vi "Map Table.vi"(8 "error in":errorcluster, 9 "Inital Index":i32=1, 11 "picture":refnum<vi>) -> (0 "error out":errorcluster, 5 "picture":picture)   [LabVIEW 2013]
uses:
  Baxter Examples/Arm Globals.vi
  ROS/Code/SubVIs/BaxterSide.ctl
  Prim/Fwd Kenimatics - array.vi
  <vilib>/Analysis/Matrix/NI_Matrix.lvlib
  <vilib>/Analysis/Matrix/Numeric/Multiply/Multiply - RM,RM.vi
  <vilib>/Analysis/Matrix/Datatypes/RealMatrix.ctl
  <vilib>/Analysis/NI_AALBase.lvlib
  <vilib>/Analysis/baseanly.llb/Mean (DBL).vi
  Move Relative XYZRPY.vi
panel:
  # "0:Far Left\n1:Far Right\n2:Near Left\n3:Near Right"
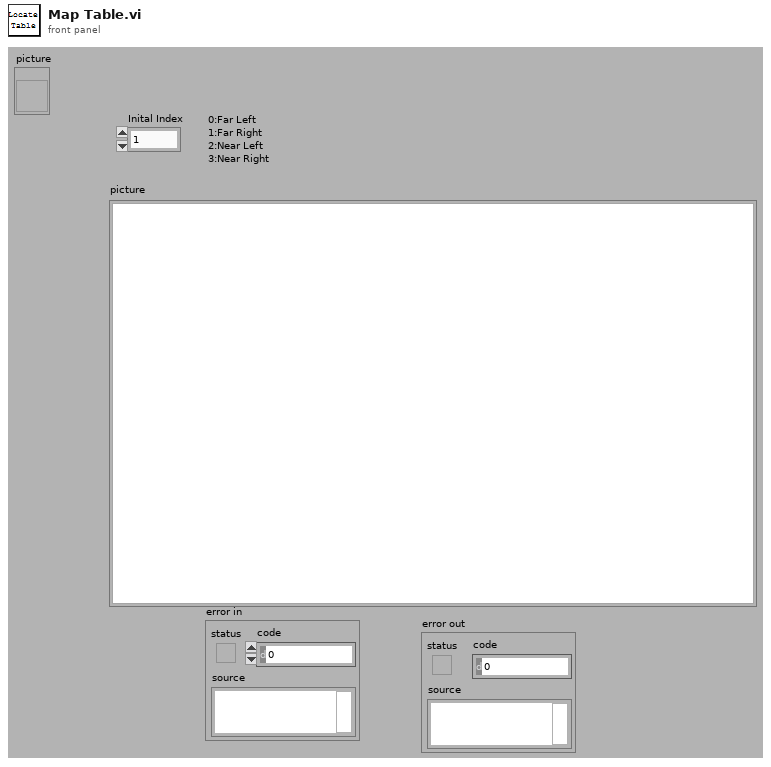
[diagram p1: front panel]
types:
  T1 = typedef "NI_Matrix.lvlib/RealMatrix.ctl" = dbl[][]
  T2 = cluster{"Label":string, "Joints":dbl[], "T":T1}[]
  T3 = typedef "BaxterSide.ctl" = enum16{"left", "right"}
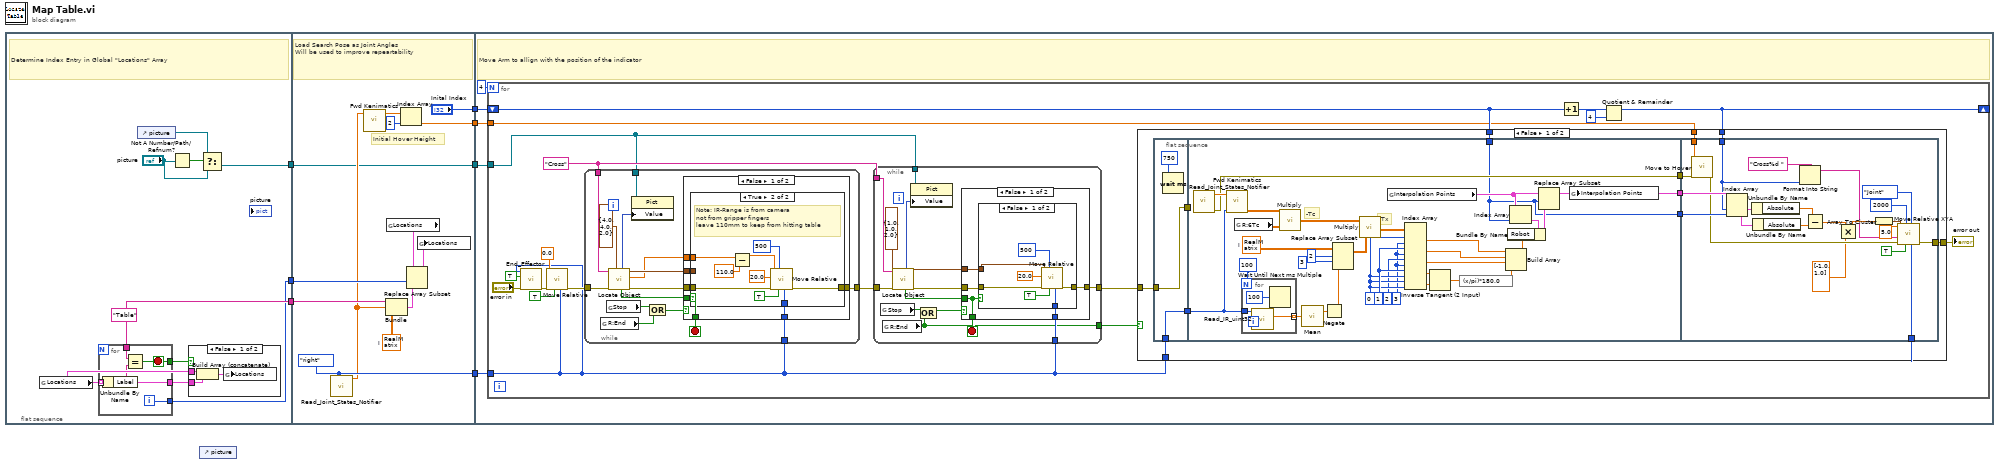
[diagram p0: block diagram]
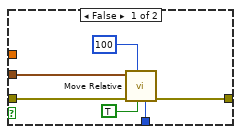
[diagram p6: hidden frame]
diagram:
  n1 = flat-sequence {
    tunnel: [w14] -> w6
    tunnel: [w16] -> w5
    tunnel: [w8] -> w1
    tunnel: [w37] -> w7
    tunnel: w6 -> [w28]
    tunnel: w5 -> [w27]
    tunnel: ["Inital Index"] -> w4
    tunnel: [w33] -> w3
    tunnel: [w25] -> w2
    tunnel: w1 -> [w25]
    tunnel: w7 -> [w42]
    tunnel: w4 -> [w40]
    tunnel: w3 -> [w39]
    tunnel: w2 -> [w38]
    frame #0 {
      w16 = "Table"
      # "Determine Index Entry in Global \"Locations\" Array"
      n2 = global read "Arm Globals.vi" "Locations"() -> (w12:T2)
      n3 = for {
        tunnel: w12 -> [w20] mode=indexing
        tunnel: w16 -> [w23]
        tunnel: [w22] -> w14
        tunnel: [w21] -> w15
        tunnel: [w20] -> w13
        i -> [w22]
        stop <- w21 stop-if-true
        n4 = Unbundle By Name(w20) -> ("Label"=w24:string)
        n5 = Equal?(x=w23, y=w24) -> (x = y?=w21:bool)
      }
      n6 = control-ref of="picture"() -> (w9:refnum<vi>)
      n7 = Not A Number/Path/Refnum?(number/path/refnum="picture") -> (NaN/Path/Refnum?=w11:bool)
      n8 = case shown="False" w15 {
        tunnel: w13 -> [w18 _]
        tunnel: w12 -> [w17 _]
        frame False {
          n9 = Build Array (concatenate)(w17, w18) -> (w19:T2)
          n10 = global write "Arm Globals.vi" "Locations"(w19) -> ()
        }
        frame True {
        }
      }
      n11 = Select(t=w9, s=w11, f="picture") -> (s? t:f=w8:refnum<vi>)
    }
    frame #1 {
      w31 = T1 [[1.0, 0.0, 0.0, 0.0], [0.0, 1.0, 0.0, 0.0], [0.0, 0.0, 1.0, 0.0], [0.0, 0.0, 0.0, 1.0]]  # I
      w37 = BaxterSide."right" ("Side")
      # "Initial Hover Height"
      # "Load Search Pose as Joint Angles\nWill be used to improve repeartability"
      n12 = call "Read_Joint_States_Notifier.vi"("Side"=w37) -> ("Positions"=w26:dbl[])  [unwired: 6 in, 1 out]
      n13 = call-poly "Fwd Kenimatics.vi"("Joints"=w26) -> ("Position"=w35:dbl[])  [unwired: 9 in, 1 out]
      n14 = Bundle(w27, "Positions"=w26, "I"=w31) -> (w32:cluster{string, "Positions":dbl[], "I":T1})  [unwired: 1 in]
      n15 = global read "Arm Globals.vi" "Locations"() -> (w30:T2)
      n16 = Index Array(array=w35, index=2) -> (element=w33:dbl)
      n17 = Replace Array Subset(array=w30, new element=w32, index=w28) -> (w29:T2)
      n18 = global write "Arm Globals.vi" "Locations"(w29) -> ()
    }
    frame #2 {
      # "Move Arm to allign with the position of the indicator"
      n19 = for {
        N: 4 -> [_]
        tunnel: w42 -> [w46]
        shift-right: [w47] -> _
        shift-left: w40 -> [w49]
        tunnel: w39 -> [w48]
        tunnel: w38 -> [w44]
        w55 = "Cross"
        n20 = call "End_Effector.vi"("error in"="error in", "Open"=TRUE, "Side"=w46) -> ("error out"=w58:errorcluster)  [unwired: 5 in]
        n21 = call-poly "Move Relative.vi"("Side"=w46, "Make Vertical"=TRUE, "error in"=w58, "Label"=0.0 ("Z")) -> ("error out"=w57:errorcluster)  [unwired: 7 in]
        n22 = while {
          tunnel: w57 -> [w176]
          tunnel: [w174] -> w60
          tunnel: w55 -> [w171]
          tunnel: w46 -> [w170]
          tunnel: w44 -> [w165]
          stop <- w168 stop-if-true
          n23 = global read "Arm Globals.vi" "R:End"() -> (w166:bool)
          n24 = global read "Arm Globals.vi" "Stop"() -> (w172:bool)
          n25 = call "Locate Object.vi"("Tolerance"=cluster{"x":dbl, "y":dbl, "a":dbl} {"x"=4.0, "y"=4.0, "a"=2.0}, "error in"=w176, "Object"=w171) -> ("error out"=w175:errorcluster, "Range"=w162:dbl, "result"=w173:cluster{"x":dbl, "y":dbl, "a":dbl}, "Close"=w167:bool, "picture"=w163:picture)  [unwired: 3 in, 1 out]
          n26 = property class="Pict"(reference=w165, "Value"=w163) -> ()  [unwired: 1 in, 2 out]
          n27 = Compound Arithmetic op=OR(w172, w166) -> (w169:bool)
          n28 = case shown="False" w169 {
            selector: w169 -> [_ w198]
            tunnel: w175 -> [w182 w199]
            tunnel: [w181 w199] -> w174
            tunnel: w173 -> [w180 _]
            tunnel: w170 -> [w179 _]
            tunnel: [w178 w198] -> w168
            tunnel: w167 -> [w178 _]
            tunnel: w162 -> [w177 _]
            frame False {
              n29 = case shown="True" w178 {
                tunnel: w182 -> [w188 w196]
                tunnel: [w187 w195] -> w181
                tunnel: w180 -> [w184 _]
                tunnel: w179 -> [w186 w194]
                tunnel: w177 -> [_ w190]
                frame False {
                  n30 = call-poly "Move Relative.vi"("Side"=w186, "Make Vertical"=TRUE, "wait time"=100, "error in"=w188, "Goal"=w184) -> ("error out"=w187:errorcluster)  [unwired: 6 in]
                }
                frame True {
                  # "Note: IR-Range is from camera \nnot from gripper fingers\nleave 110mm to keep from hitting table"
                  n31 = Subtract(x=w190, y=110.0) -> (x-y=w189:dbl)
                  n32 = call-poly "Move Relative.vi"("Side"=w194, "Make Vertical"=TRUE, "wait time"=500, "error in"=w196, "Label"=20.0 ("Speed"), "XYZOAT"=w189) -> ("error out"=w195:errorcluster)  [unwired: 5 in]
                }
              }
            }
            frame True {
            }
          }
        }
        n33 = while {
          tunnel: w60 -> [w146]
          tunnel: [w144] -> w52
          tunnel: w55 -> [w141]
          tunnel: w46 -> [w140]
          tunnel: w44 -> [w136]
          tunnel: [w133] -> w43
          stop <- w137 stop-if-true
          n34 = global read "Arm Globals.vi" "Stop"() -> (w142:bool)
          n35 = global read "Arm Globals.vi" "R:End"() -> (w133:bool)
          n36 = call "Locate Object.vi"("Tolerance"=cluster{"x":dbl, "y":dbl, "a":dbl} {"x"=1.0, "y"=1.0, "a"=2.0}, "error in"=w146, "Object"=w141) -> ("error out"=w145:errorcluster, "result"=w143:cluster{"x":dbl, "y":dbl, "a":dbl}, "Close"=w138:bool, "picture"=w134:picture)  [unwired: 3 in, 2 out]
          n37 = property class="Pict"(reference=w136, "Value"=w134) -> ()  [unwired: 1 in, 2 out]
          n38 = Compound Arithmetic op=OR(w142, w133) -> (w139:bool)
          n39 = case shown="False" w139 {
            selector: w139 -> [_ w160]
            tunnel: w138 -> [w147 _]
            tunnel: w145 -> [w151 w161]
            tunnel: [w150 w161] -> w144
            tunnel: w143 -> [w149 _]
            tunnel: w140 -> [w148 _]
            tunnel: [w147 w160] -> w137
            frame False {
              n40 = case shown="False" w147 {
                tunnel: w151 -> [w158 w159]
                tunnel: [w157 w159] -> w150
                tunnel: w149 -> [w154 _]
                tunnel: w148 -> [w156 _]
                frame False {
                  n41 = call-poly "Move Relative.vi"("Side"=w156, "Make Vertical"=TRUE, "wait time"=500, "error in"=w158, "Label"=20.0 ("Speed"), "XYZOAT"=w154) -> ("error out"=w157:errorcluster)  [unwired: 5 in]
                }
                frame True {
                }
              }
            }
            frame True {
            }
          }
        }
        n42 = Increment(x=w49) -> (x+1=w51:i32)
        n43 = Quotient & Remainder(x=w51, y=4) -> (x-y*floor(x/y)=w47:i32)  [unwired: 1 out]
        n44 = case shown="False" w43 {
          tunnel: w52 -> [w66 w132]
          tunnel: w49 -> [w65 _]
          tunnel: w48 -> [w64 _]
          tunnel: w47 -> [w63 _]
          tunnel: w46 -> [w62 _]
          tunnel: [w61 w132] -> w45
          frame False {
            n45 = flat-sequence {
              tunnel: w66 -> [w74]
              tunnel: w62 -> [w73]
              tunnel: [w74] -> w71
              tunnel: [w73] -> w70
              tunnel: w71 -> [_]
              tunnel: w70 -> [w78]
              tunnel: w65 -> [w75]
              tunnel: [w77] -> w69
              tunnel: [w76] -> w68
              tunnel: [w75] -> w67
              tunnel: w64 -> [w131]
              tunnel: w69 -> [w130]
              tunnel: w68 -> [w128]
              tunnel: w63 -> [w118]
              tunnel: w67 -> [w127]
              tunnel: w62 -> [w122]
              tunnel: [w119] -> w61
              frame #0 {
                n46 = Wait (ms)(milliseconds to wait=u32 750) -> ()  [unwired: 1 out]
              }
              frame #1 {
                w97 = 1 ("index (row)")
                w92 = 3 ("index (col)")
                w96 = 0 ("index (row)")
                w86 = T1 [[1.0, 0.0, 0.0, 0.0], [0.0, 1.0, 0.0, 0.0], [0.0, 0.0, 1.0, 0.0], [0.0, 0.0, 0.0, 1.0]]  # I
                # "-Tx"
                # "-Tc"
                n47 = call "Read_Joint_States_Notifier.vi"() -> ("error out"=w77:errorcluster, "Positions"=w79:dbl[])  [unwired: 7 in]
                n48 = call-poly "Fwd Kenimatics.vi"("Side"=w78, "Joints"=w79) -> ("Matrix"=w82:T1)  [unwired: 8 in, 1 out]
                n49 = global read "Arm Globals.vi" "R:6Tc"() -> (w81:T1)
                n50 = for {
                  N: 100 -> [_]
                  tunnel: w78 -> [w109]
                  tunnel: [w108] -> w84 mode=indexing
                  n51 = call "Read_IR_uint32.vi"("Side"=w109) -> ("Distance"=w108:dbl)  [unwired: 4 in, 3 out]
                  n52 = Wait Until Next ms Multiple(millisecond multiple=u32 100) -> ()  [unwired: 1 out]
                }
                n53 = call-poly <vilib>:"Multiply.vi"("Real Matrix B"=w81, "Real Matrix A"=w82) -> ("A * B"=w89:T1)
                n54 = call-poly <vilib>:"Mean.vi"("X"=w84) -> ("mean"=w83:dbl)  [unwired: 1 out]
                n55 = Negate(x=w83) -> (-x=w88:dbl)
                n56 = Replace Array Subset(array=w86, new element=w88, index (row)=2 ("disabled index (row)"), index (col)=3 ("disabled index (col)")) -> (w90:T1)
                n57 = call-poly <vilib>:"Multiply.vi"("Real Matrix B"=w90, "Real Matrix A"=w89) -> ("A * B"=w91:T1)
                n58 = global read "Arm Globals.vi" "Interpolation Points"() -> (w105:cluster{"Absolute":dbl[], "Robot":dbl[]}[])
                n59 = Index Array(array=w91, index (row) #1=w96, index (col) #1=w92, index (row) #2=w97, index (col) #2=w92, index (row) #3=2 ("index (row)"), index (col) #3=w92, index (row) #4=w97, index (col) #4=w96, index (row) #5=w96, index (col) #5=w96) -> (element #1=w102:dbl, element #2=w101:dbl, element #3=w100:dbl, element #4=w94:dbl, element #5=w95:dbl)
                n60 = Inverse Tangent (2 Input)(1:w95, 2:w94) -> (0:w98:dbl)
                n61 = expression code="(x/pi)*180.0" ("radians to degrees")(w98) -> (w99:dbl)
                n62 = Build Array(w102, w101, w100, w99) -> (w104:dbl[])
                n63 = Index Array(array=w105, index=w75) -> (element=w103:cluster{"Absolute":dbl[], "Robot":dbl[]})
                n64 = Bundle By Name(cluster=w103, "Robot"=w104) -> (w106:cluster{"Absolute":dbl[], "Robot":dbl[]})
                n65 = Replace Array Subset(array=w105, new element=w106, index=w75) -> (w76:cluster{"Absolute":dbl[], "Robot":dbl[]}[])
                n66 = global write "Arm Globals.vi" "Interpolation Points"(w76) -> ()
              }
              frame #2 {
                n67 = call "Move to Hover.vi"("error in"=w130, "Z"=w131) -> ("error out"=w120:errorcluster)  [unwired: 9 in]
                n68 = Index Array(array=w128, index #1=w118, index #2=w127) -> (element #1=w129:cluster{"Absolute":dbl[], "Robot":dbl[]}, element #2=w126:cluster{"Absolute":dbl[], "Robot":dbl[]})
                n69 = Unbundle By Name(w129) -> ("Absolute"=w125:dbl[])
                n70 = Unbundle By Name(w126) -> ("Absolute"=w124:dbl[])
                n71 = Format Into String(format string="Cross%d ", w118) -> (resulting string=w111:string)  [unwired: 2 in, 1 out]
                n72 = Subtract(x=w125, y=w124) -> (x-y=w115:dbl[])
                n73 = Multiply(x=w115, y=dbl[] [-1.0, 1.0]) -> (x*y=w114:dbl[])
                n74 = Array To Cluster(array=w114) -> (cluster=w123:cluster{"[0]":dbl, "[1]":dbl, "[2]":dbl})
                n75 = call "Move Relative XYA.vi"("Side"=w122, "Motion"=enum16{"Joint", "Linear"}."Joint", "Make Vertical"=TRUE, "wait time"=2000, "error in"=w120, "Speed"=w111, "Label"=5.0 ("Speed"), "Goal"=w123) -> ("error out"=w119:errorcluster)  [unwired: 3 in]
              }
            }
          }
          frame True {
          }
        }
        "error out" <- w45
      }
    }
  }
  n76 = control-ref of="picture"() -> ()  [unwired: 1 out]
